vi "Assignment 2.vi"() -> ()   [LabVIEW 2024]
panel:
  out "K 2":dbl
  in  "F 2":dbl
  out "K 1":dbl
  in  "F 1":dbl
  out "A2 Total":dbl
  out "A1 Total":dbl
  out "B2":dbl
  out "B1":dbl
  in  "C2":dbl
  in  "A2":dbl
  in  "C1":dbl
  in  "A1":dbl
  out "TOAL Square Root 2":dbl
  out "TOTAL Square 2":dbl
  out "TOAL Square Root":dbl
  out "TOTAL Square":dbl
  in  "X2":dbl
  in  "X":dbl
  # "Pythagorean Theorem"
  # "Square/ Square Root"
  # "Fahrenheit to Kelvin"
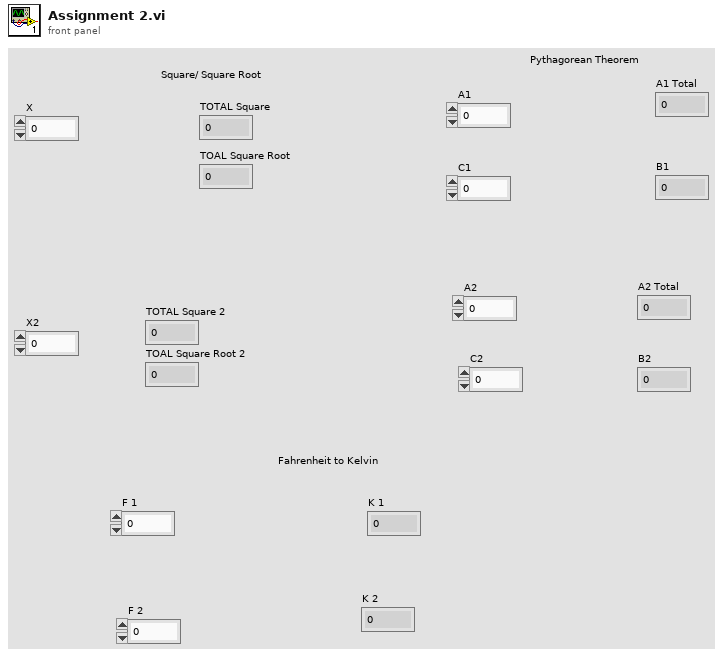
[diagram p1: front panel]
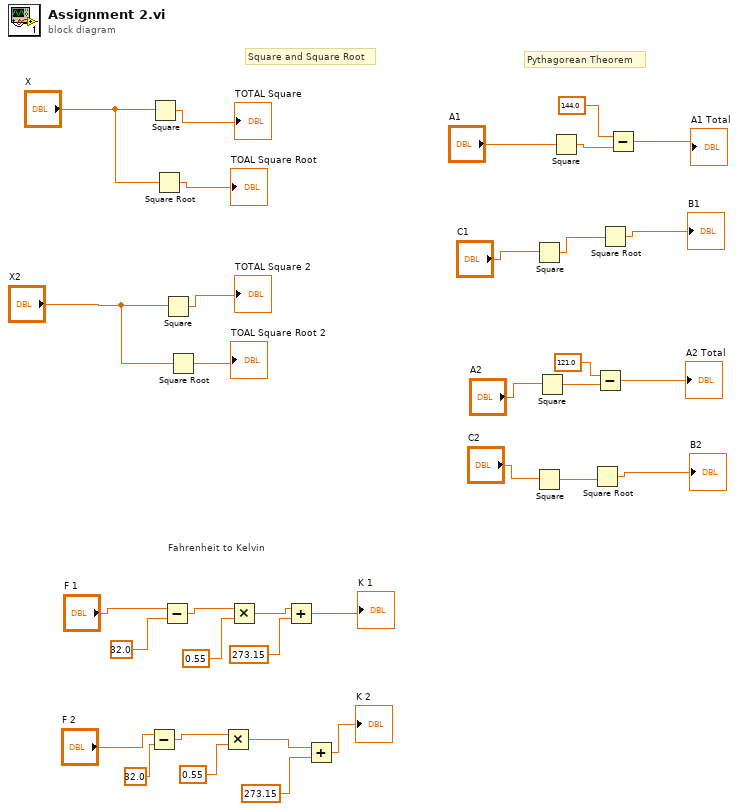
[diagram p0: block diagram]
diagram:
  # "Fahrenheit to Kelvin"
  # "Pythagorean Theorem"
  # "Square and Square Root"
  n1 = Subtract(x="F 2", y=32.0) -> (x-y=w8:dbl)
  n2 = Square(x="X") -> (x^2=→"TOTAL Square":dbl)
  n3 = Square Root(x="X") -> (sqrt(x)=→"TOAL Square Root":dbl)
  n4 = Subtract(x="F 1", y=32.0) -> (x-y=w7:dbl)
  n5 = Square(x="X2") -> (x^2=→"TOTAL Square 2":dbl)
  n6 = Square Root(x="X2") -> (sqrt(x)=→"TOAL Square Root 2":dbl)
  n7 = Multiply(x=w8, y=0.55) -> (x*y=w6:dbl)
  n8 = Multiply(x=w7, y=0.55) -> (x*y=w5:dbl)
  n9 = Add(x=w5, y=273.15) -> (x+y=→"K 1":dbl)
  n10 = Add(x=w6, y=273.15) -> (x+y=→"K 2":dbl)
  n11 = Square(x="C1") -> (x^2=w23:dbl)
  n12 = Square(x="C2") -> (x^2=w16:dbl)
  n13 = Square(x="A2") -> (x^2=w20:dbl)
  n14 = Square(x="A1") -> (x^2=w27:dbl)
  n15 = Square Root(x=w16) -> (sqrt(x)=→"B2":dbl)
  n16 = Subtract(x=121.0, y=w20) -> (x-y=→"A2 Total":dbl)
  n17 = Square Root(x=w23) -> (sqrt(x)=→"B1":dbl)
  n18 = Subtract(x=144.0, y=w27) -> (x-y=→"A1 Total":dbl)
